vi "Actor Core.vi"(8 "error in":errorcluster, 11 "ViewableLaunchesDialogBox In":refnum<class "ViewableLaunchesDialogBox.lvclass">) -> (0 "error out":errorcluster, 3 "Actor out":refnum<class "Actor.lvclass">)   [LabVIEW 2018, in "ViewableLaunchesDialogBox.lvclass"]
doc: "(<B>Filename</B>: Actor Framework.lvlib:Actor.lvclass:Actor Core.vi)\n\nReceives messages to the actor, reacts to them, and initiates any error handling that may shut the actor down.\n\nDescendant classes may override this VI to append parallel tasks for the actor to complete while it handles messages. Overrides use the Call Parent Method node.\n\n<License>\nCopyright © 2017 Composed Systems, LLC | All rights reserved\nwww.composed.io\n\nAuthor: Ethan Stern <ethan.stern@composed.io>\n\nThis software is provided \"AS IS\" WITHOUT WARRANTIES, either express or implied, AND IS FOR EDUCATIONAL PURPOSES ONLY.\n</License>"
uses:
  ViewableLaunchesDialogBox.lvclass
  Source/IDialogBox/IDialogBox/IDialogBox.lvclass
  modules/mva-viewable/Source/IViewable/IViewable/IViewable.lvclass
  <vilib>/ActorFramework/Actor/Actor.lvclass
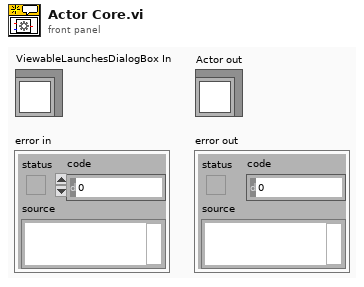
[diagram p1: front panel]
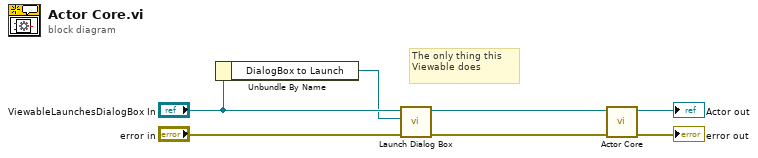
[diagram p0: block diagram]
diagram:
  # "The only thing this\nViewable does"
  n1 = Unbundle By Name("ViewableLaunchesDialogBox In") -> ("DialogBox to Launch"=w2:refnum<class "IDialogBox.lvclass">)
  n2 = call "Launch Dialog Box.vi"("error in (no error)"="error in", "DialogBox"=w2, "DialogBox Launcher"="ViewableLaunchesDialogBox In") -> ("error out"=w1:errorcluster, "DialogBox Launcher Out"=w4:refnum<class "ViewableLaunchesDialogBox.lvclass">)  [unwired: 6 in, 1 out]
  n3 = call-parent "Actor Core.vi"("error in"=w1, "IViewable In"=w4) -> ("error out"=→"error out":errorcluster, "Actor out"=→"Actor out":refnum<class "Actor.lvclass">)  [unwired: 8 in]
